vi "参数配置表.vi"() -> ()   [LabVIEW 2016, in "数据传输系统-03.lvlib"]
uses:
  <vilib>/Utility/miscctls.llb/LVPointTypeDef.ctl
  <vilib>/ptbypt/NI_PtbyPt.lvlib
panel:
  in  "参数数值":T1={"CODMn"=TRUE, "CODCr"=TRUE, "DO"=TRUE, "铜"=TRUE, "PH"=TRUE, "氨氮"=TRUE, "比电导率"=TRUE, "水温"=TRUE, "COD"=TRUE, "浊度"=TRUE, "总氮"=TRUE, "总磷"=TRUE, "叶绿素a"=TRUE, "藻密度"=TRUE, "水位"=TRUE, "流速"=TRUE, "方向"=TRUE, "瞬时流量"=TRUE, "累积流量"=TRUE, "正累积流量"=TRUE, "负累积流量"=TRUE, "亚硝氮"=TRUE, "硫化物"=TRUE, "ORP"=TRUE, "铅"=TRUE, "镉"=TRUE, "锌"=TRUE, "镍"=TRUE, "锰"=TRUE, "汞"=TRUE, "气温"=TRUE, "气压"=TRUE, "风速"=TRUE, "风向"=TRUE, "空气温度"=TRUE, "相对湿度"=TRUE, "分钟雨量"=TRUE, "小时雨量"=TRUE, "日雨量"=TRUE, "累积雨量"=TRUE, "盐度"=TRUE, "磷酸盐"=TRUE, "硝氮"=TRUE, "氟化物"=TRUE, "挥发酚"=TRUE, "氯化物"=TRUE, "蓝绿藻"=TRUE, "余氯"=TRUE, "综合生物毒性"=TRUE, "艏向"=TRUE, "横摇"=TRUE, "纵摇"=TRUE, "分层标志"=TRUE, "层状态1"=TRUE, "层状态2"=TRUE, "水平平均流速"=TRUE, "流向"=TRUE, "北向流速分量"=TRUE, "东向流速分量"=TRUE, "垂直流速分量"=TRUE, "最大波高"=TRUE, "最大波周期"=TRUE, "1/10波高"=TRUE, "1/10波周期"=TRUE, "有效波高"=TRUE, "有效波周期"=TRUE, "平均波高"=TRUE, "平均波周期"=TRUE, "波向"=TRUE, "波个数"=TRUE, "水深"=TRUE, "X轴流速"=TRUE, "Y轴流速"=TRUE, "信号强度"=TRUE, "电压"=TRUE, "悬浮物"=TRUE}
  in  "协议标准":T2(ring)
  in  "加密传输":bool
  in  "数据库类型":enum16{"Access", "SQLite"}(ring)
  in  "应用环境":T3
  in  "屏蔽维护数据":bool
  in  "数据发送延时时间/s":i32
  in  "判断数据反馈":enum16{"非严格判断", "严格判断", "不判断"}(ring)
  in  "仪器参数发送":bool
  in  "地表水/污染源":bool
  in  "间隔时间/分钟":i32
  in  "数据发送通道":enum16{"TCP", "VISA"}(ring)
  in  "数据发送协议":enum16{"2005-212协议", "2017-212协议"}(ring)=enum."2017-212协议"
  in  "数据触发上传方式":enum16{"出数即刻发送", "间隔时间发送", "整点发送"}(ring)
  in  "数据组合发送":bool
  in  "日志、参数发送":bool
  in  "2011发送":bool
  in  "返回":bool
  out "配置表格":string[][](table)
  # "因子编码，单位配置，上传功能码，小时、质控数据上传触发方式"
  # "参数配置"
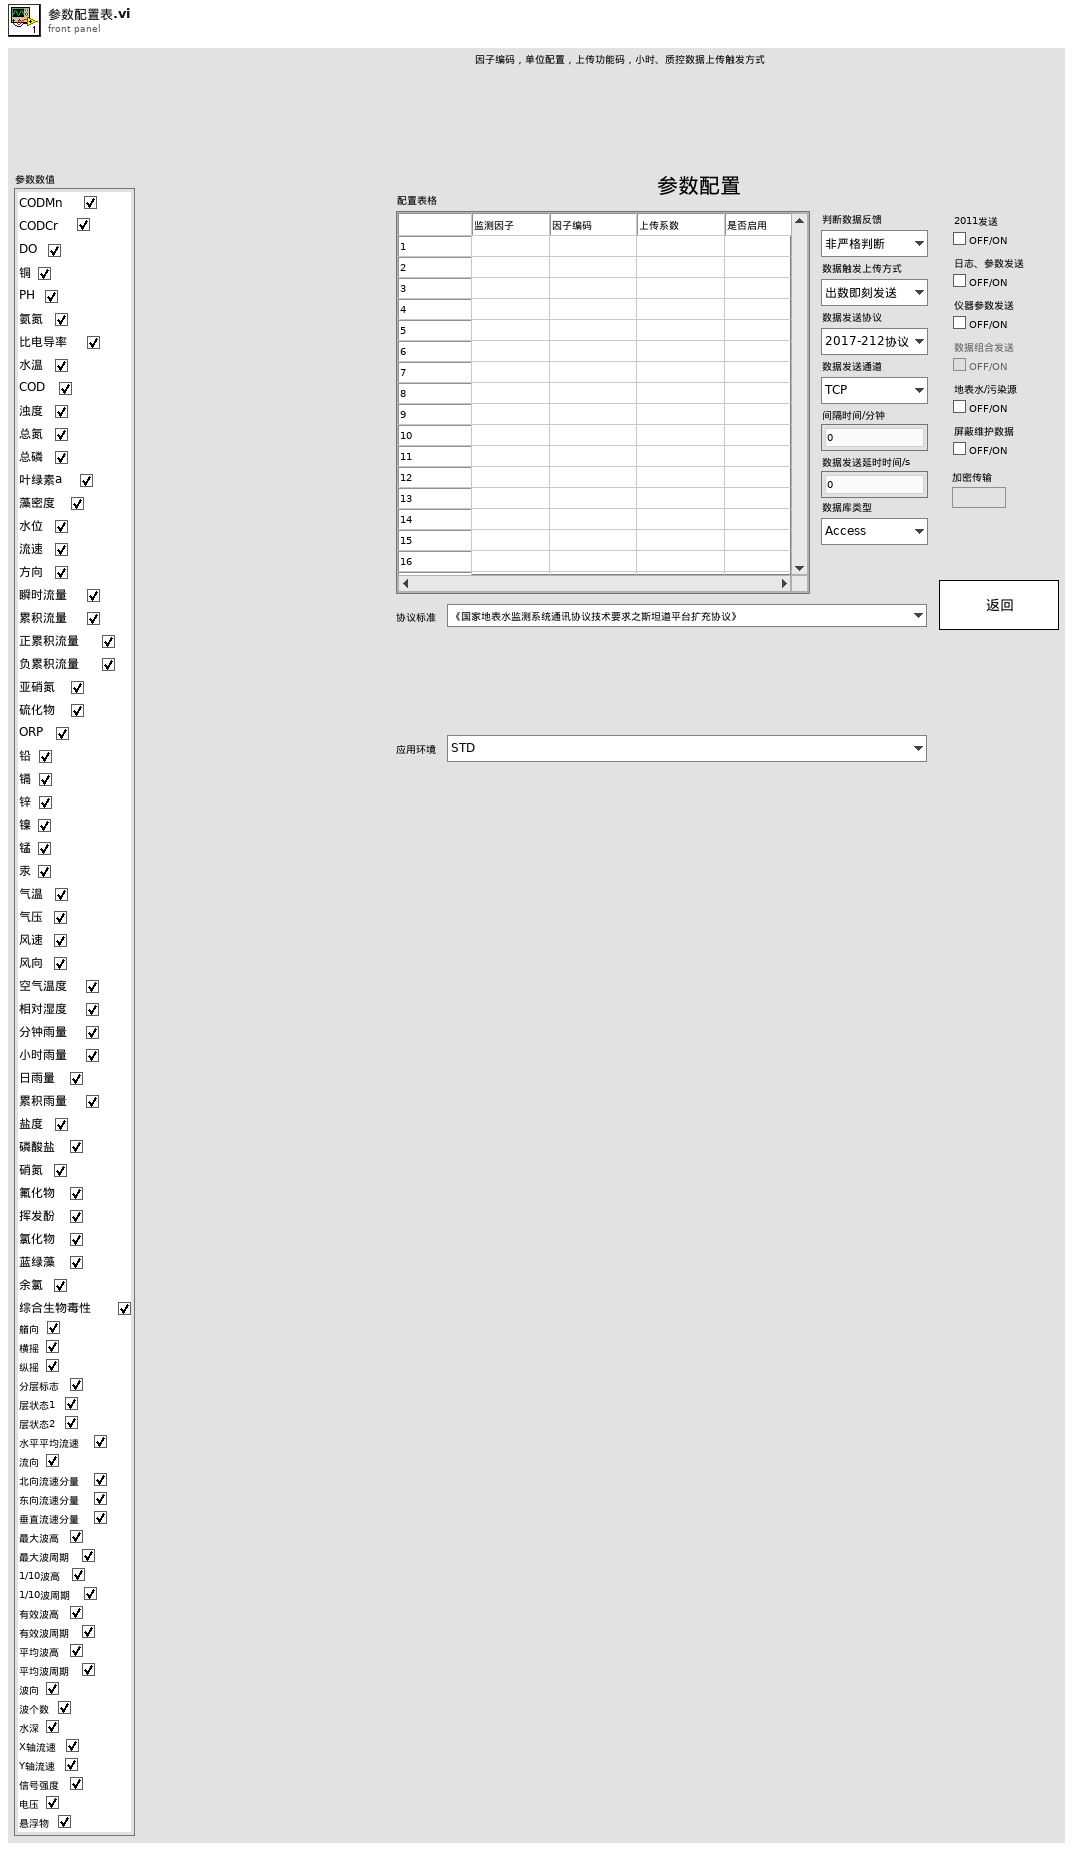
[diagram p1: front panel]
types:
  T1 = cluster{"CODMn":bool, "CODCr":bool, "DO":bool, "铜":bool, "PH":bool, "氨氮":bool, "比电导率":bool, "水温":bool, "COD":bool, "浊度":bool, "总氮":bool, "总磷":bool, "叶绿素a":bool, "藻密度":bool, "水位":bool, "流速":bool, "方向":bool, "瞬时流量":bool, "累积流量":bool, "正累积流量":bool, "负累积流量":bool, "亚硝氮":bool, "硫化物":bool, "ORP":bool, "铅":bool, "镉":bool, "锌":bool, "镍":bool, "锰":bool, "汞":bool, "气温":bool, "气压":bool, "风速":bool, "风向":bool, "空气温度":bool, "相对湿度":bool, "分钟雨量":bool, "小时雨量":bool, "日雨量":bool, "累积雨量":bool, "盐度":bool, "磷酸盐":bool, "硝氮":bool, "氟化物":bool, "挥发酚":bool, "氯化物":bool, "蓝绿藻":bool, "余氯":bool, "综合生物毒性":bool, "艏向":bool, "横摇":bool, "纵摇":bool, "分层标志":bool, "层状态1":bool, "层状态2":bool, "水平平均流速":bool, "流向":bool, "北向流速分量":bool, "东向流速分量":bool, "垂直流速分量":bool, "最大波高":bool, "最大波周期":bool, "1/10波高":bool, "1/10波周期":bool, "有效波高":bool, "有效波周期":bool, "平均波高":bool, "平均波周期":bool, "波向":bool, "波个数":bool, "水深":bool, "X轴流速":bool, "Y轴流速":bool, "信号强度":bool, "电压":bool, "悬浮物":bool}
  T2 = enum16{"《国家地表水监测系统通讯协议技术要求之斯坦道平台扩充协议》", "《国家地表水监测系统通讯协议技术要求》", "《国家地表水监测系统通讯协议技术要求之安徽皖仪省级平台扩充协议》"}
  T3 = typedef "数据传输系统-03.lvlib/应用环境.ctl" = enum16{"STD", "GB212", "婉仪平台"}
  T4 = typedef "LVPointTypeDef.ctl" = cluster{"Horizontal":i16, "Vertical":i16}
  T5 = cluster{"子数组[0]":string, "子数组[1]":string, "子数组[2]":string, "子数组[3]":string, "子数组[4]":string, "子数组[5]":string, "子数组[6]":string, "子数组[7]":string, "子数组[8]":string, "子数组[9]":string, "子数组[10]":string, "子数组[11]":string, "子数组[12]":string, "子数组[13]":string, "子数组[14]":string, "子数组[15]":string, "子数组[16]":string, "子数组[17]":string, "子数组[18]":string, "子数组[19]":string, "子数组[20]":string, "子数组[21]":string, "子数组[22]":string, "子数组[23]":string, "子数组[24]":string, "子数组[25]":string, "子数组[26]":string, "子数组[27]":string, "子数组[28]":string, "子数组[29]":string, "子数组[30]":string, "子数组[31]":string, "子数组[32]":string, "子数组[33]":string, "子数组[34]":string, "子数组[35]":string, "子数组[36]":string, "子数组[37]":string, "子数组[38]":string, "子数组[39]":string, "子数组[40]":string, "子数组[41]":string, "子数组[42]":string, "子数组[43]":string, "子数组[44]":string, "子数组[45]":string, "子数组[46]":string, "子数组[47]":string, "子数组[48]":string, "子数组[49]":string, "子数组[50]":string, "子数组[51]":string, "子数组[52]":string, "子数组[53]":string, "子数组[54]":string, "子数组[55]":string, "子数组[56]":string, "子数组[57]":string, "子数组[58]":string, "子数组[59]":string, "子数组[60]":string, "子数组[61]":string, "子数组[62]":string, "子数组[63]":string, "子数组[64]":string, "子数组[65]":string, "子数组[66]":string, "子数组[67]":string, "子数组[68]":string, "子数组[69]":string, "子数组[70]":string, "子数组[71]":string, "子数组[72]":string, "子数组[73]":string, "子数组[74]":string, "子数组[75]":string}
  T6 = enum8{"Enabled", "Disabled", "Disabled and Grayed Out"}
  T7 = typedef "LVRowAndColumnTypeDef.ctl" = cluster{"Row":i32, "Column":i32}
  T8 = cluster{"[0]":string, "[1]":string, "[2]":string, "[3]":string, "[4]":string, "[5]":string, "[6]":string, "[7]":string}
  T9 = cluster{"[0]":string, "[1]":string, "[2]":string, "[3]":string, "[4]":string, "[5]":string, "[6]":string, "[7]":string, "[8]":string, "[9]":string, "[10]":string, "[11]":string, "[12]":string, "[13]":string}
  T10 = cluster{"[0]":string, "[1]":string, "[2]":string, "[3]":string, "[4]":string, "[5]":string, "[6]":string, "[7]":string, "[8]":string, "[9]":string, "[10]":string, "[11]":string, "[12]":string, "[13]":string, "[14]":string}
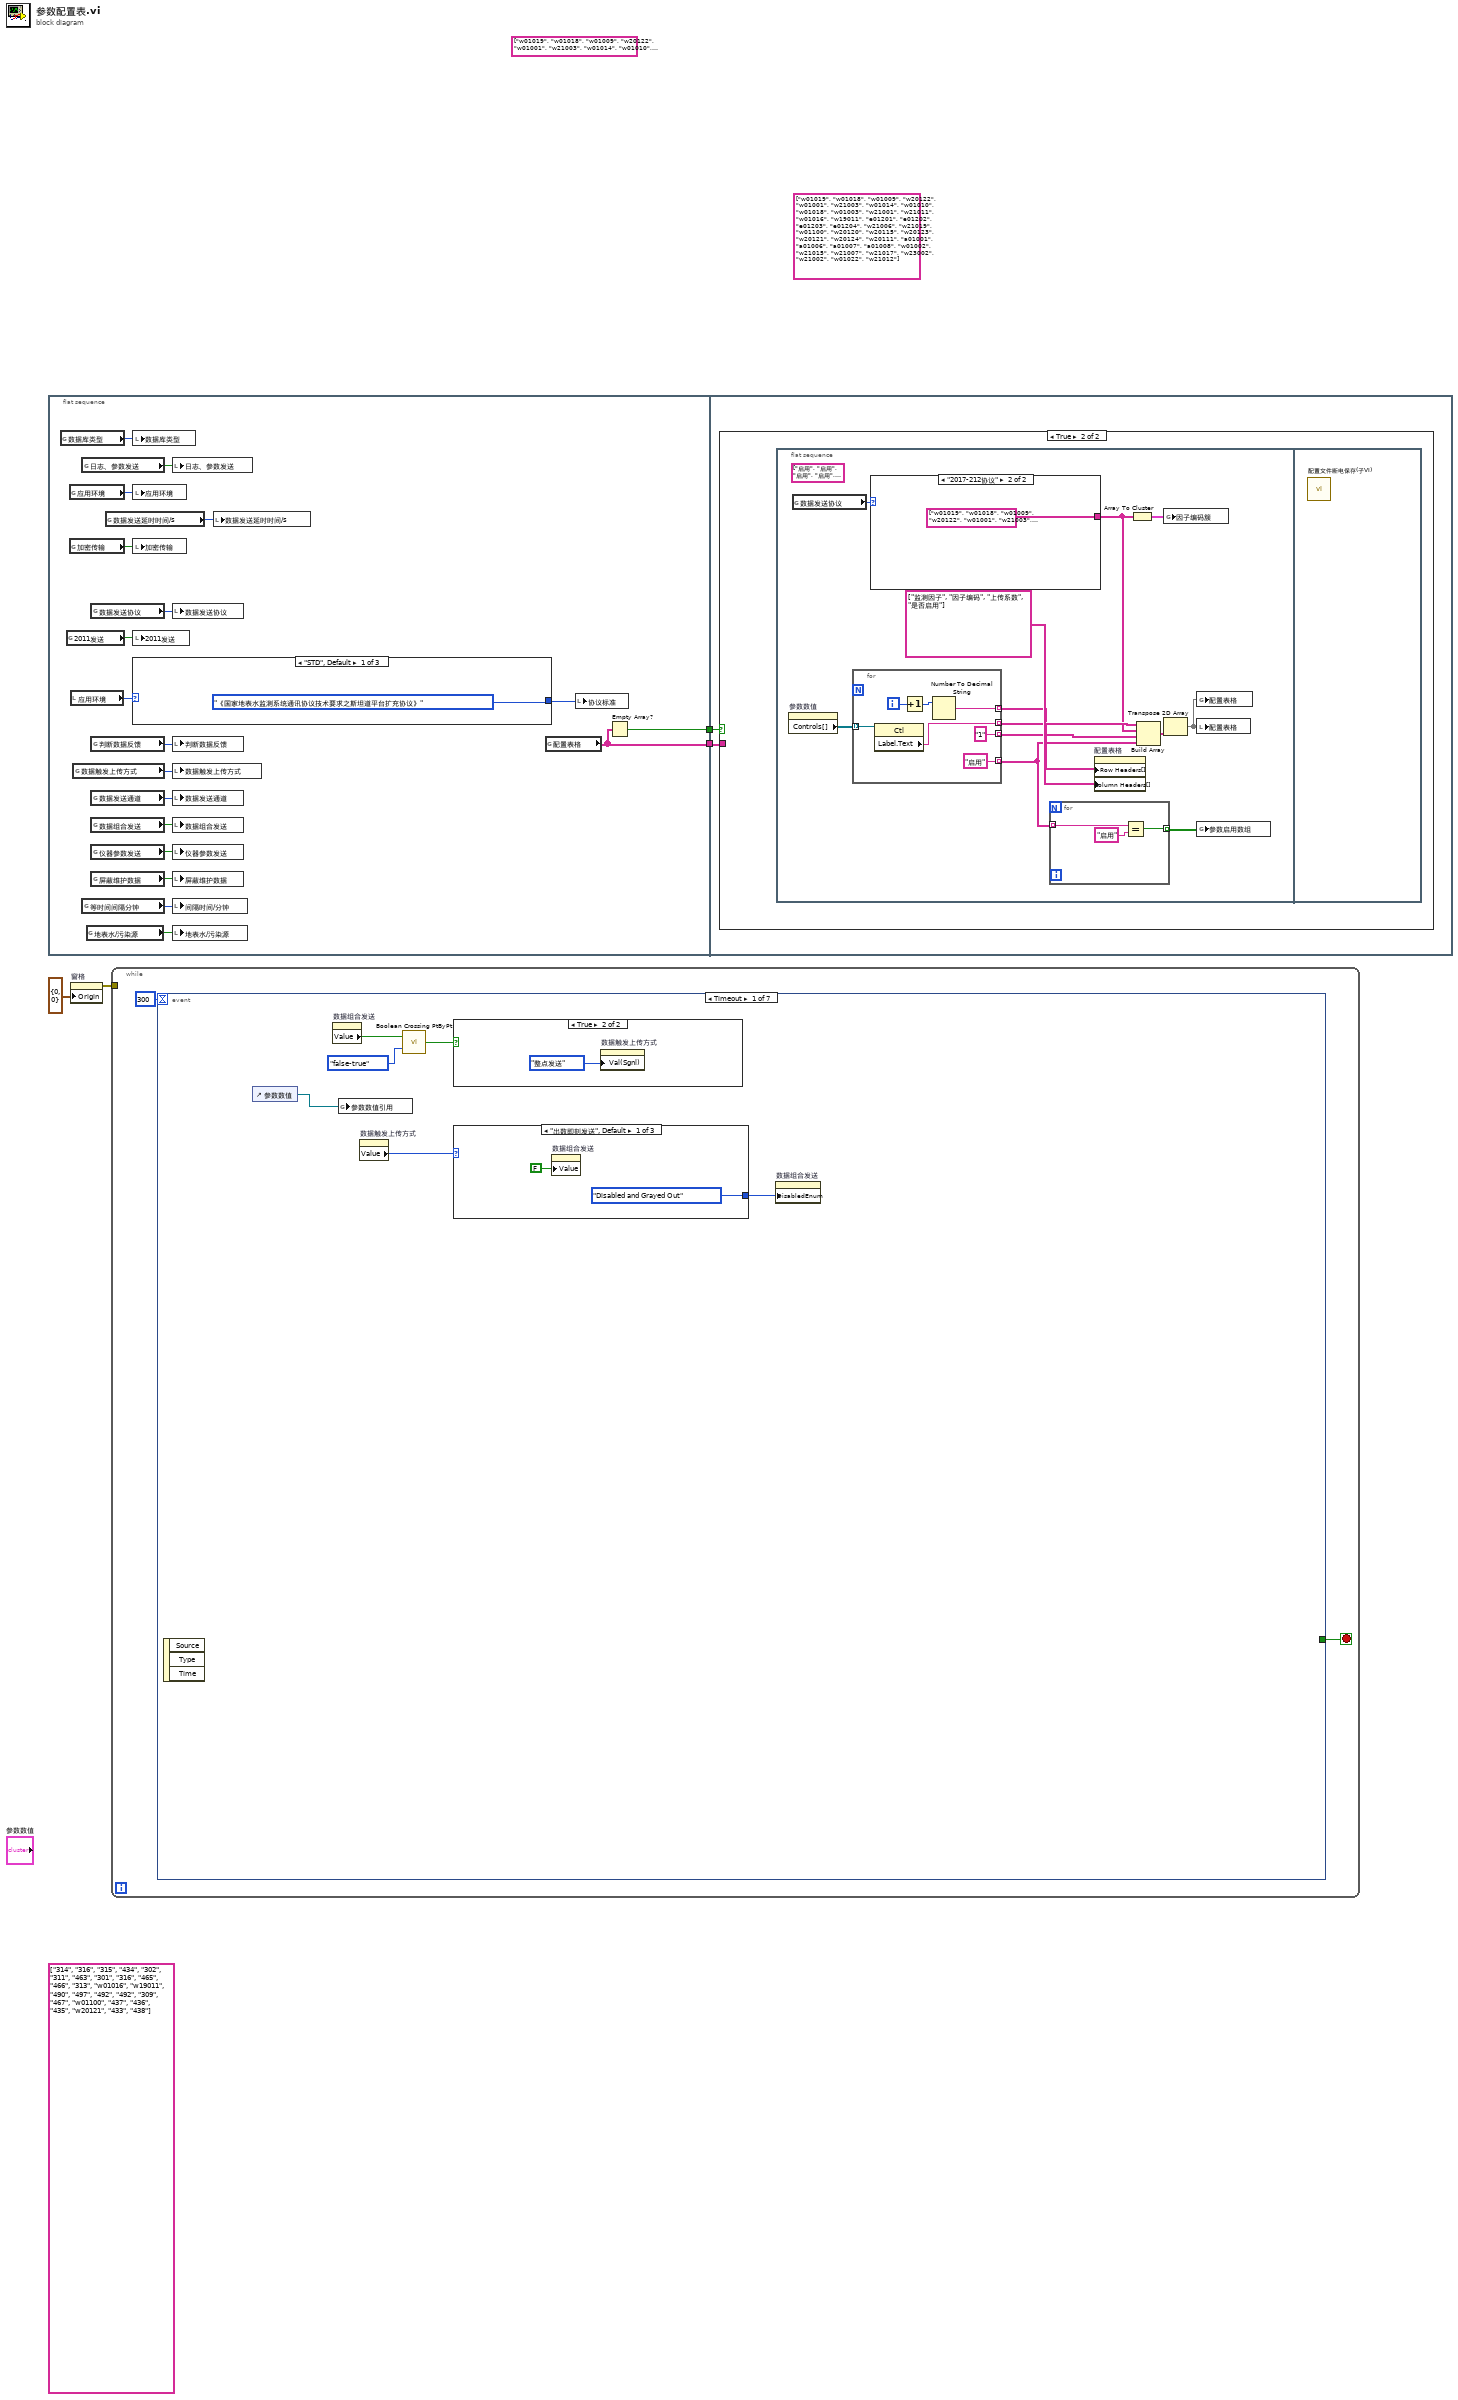
[diagram p0: block diagram]
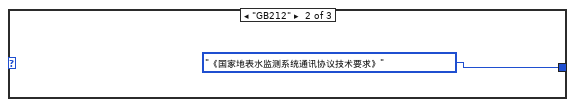
[diagram p2: hidden frame]
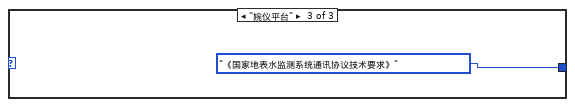
[diagram p3: hidden frame]
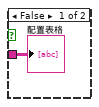
[diagram p4: hidden frame]
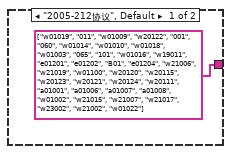
[diagram p5: hidden frame]
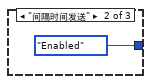
[diagram p7: hidden frame]
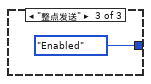
[diagram p8: hidden frame]
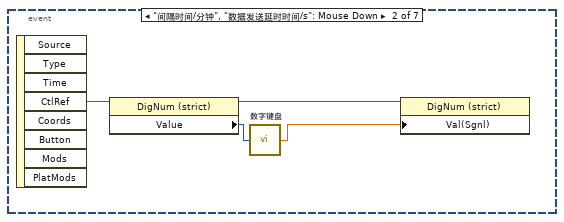
[diagram p9: hidden frame]
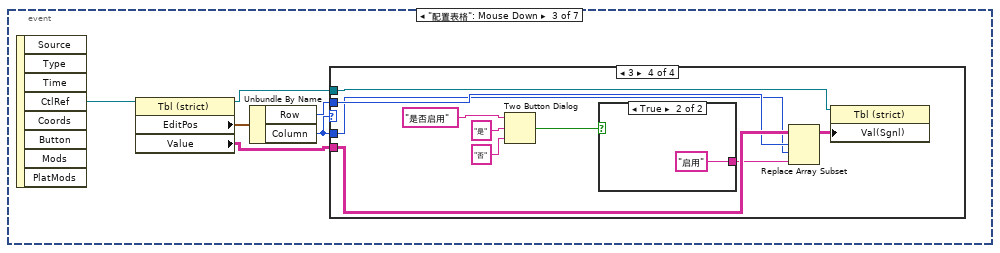
[diagram p10: hidden frame]
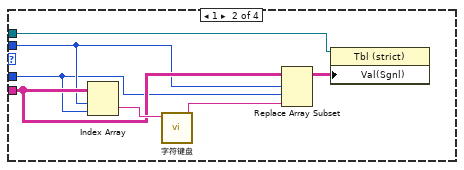
[diagram p12: hidden frame]
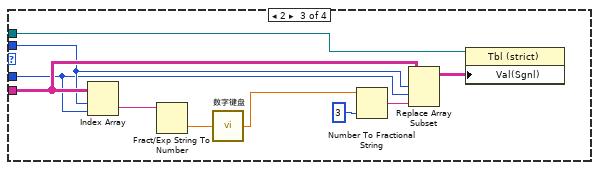
[diagram p13: hidden frame]
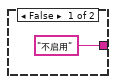
[diagram p14: hidden frame]
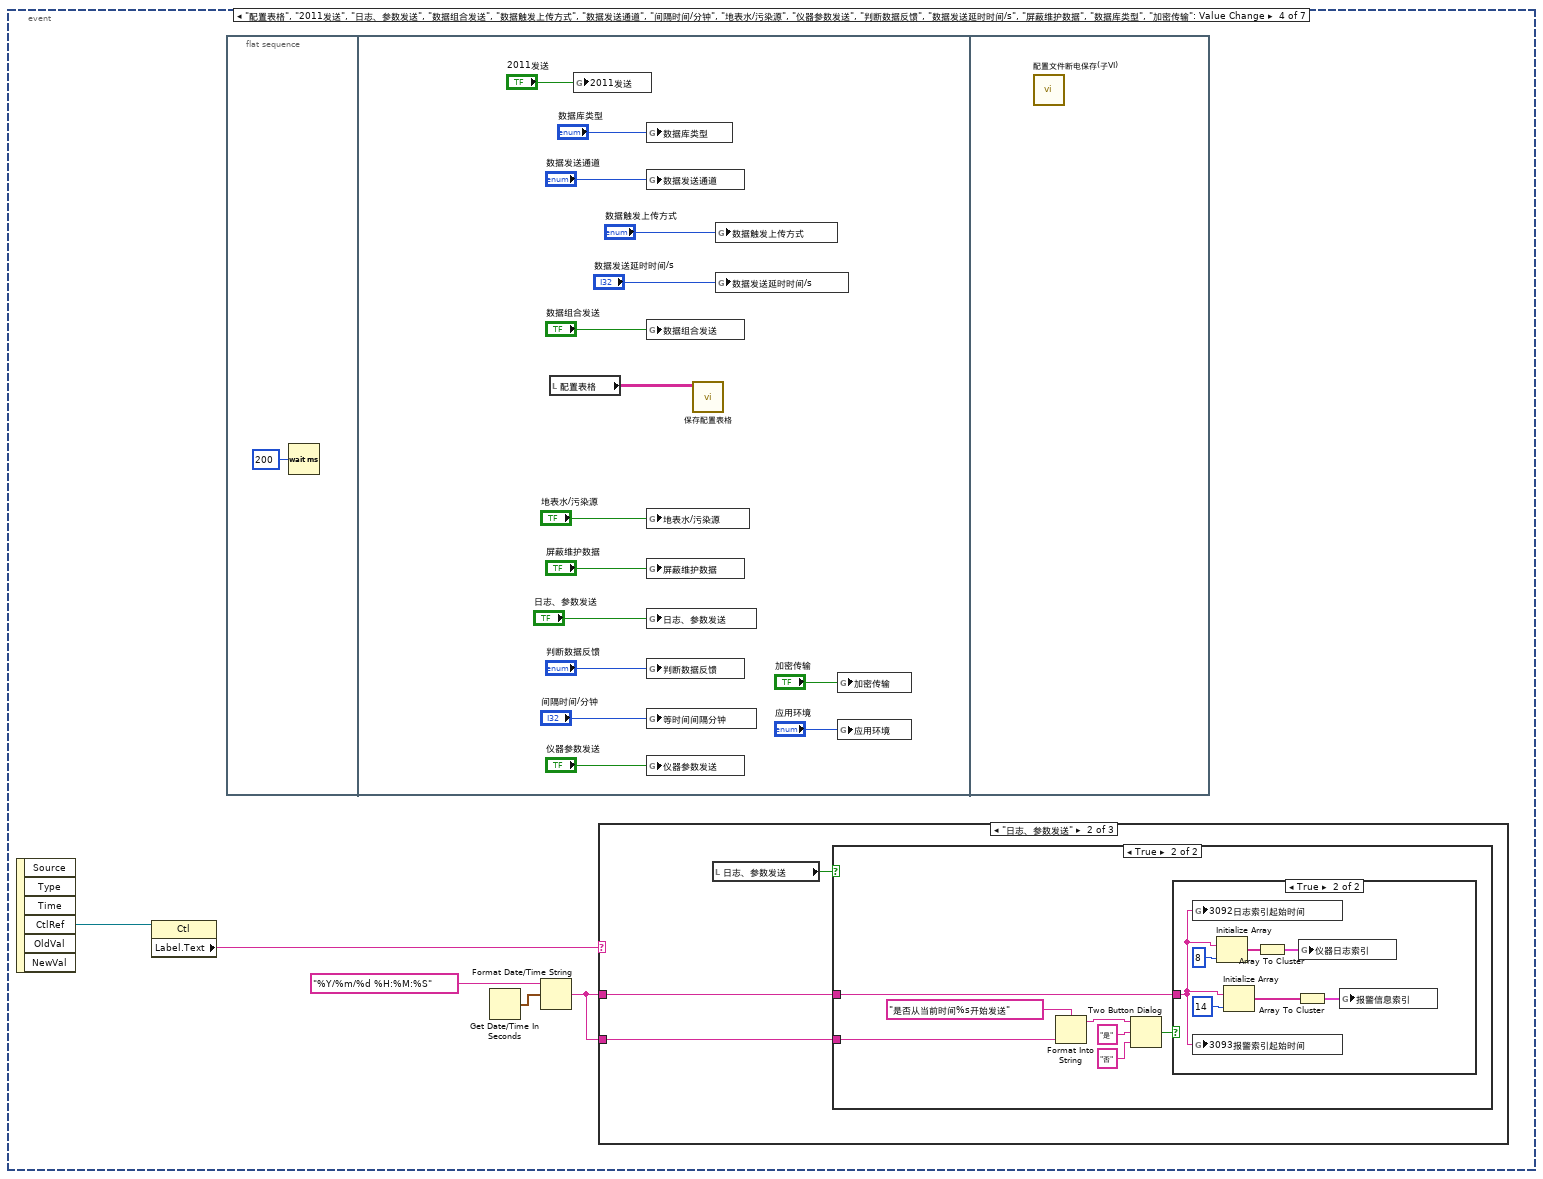
[diagram p15: hidden frame]
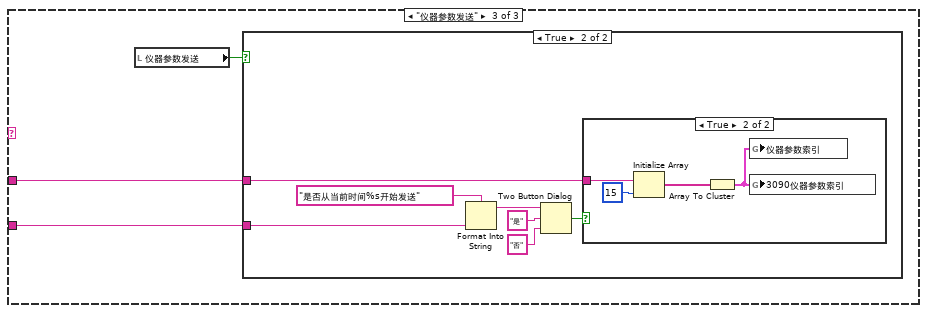
[diagram p19: hidden frame]
diagram:
  (unwired) string[] ["w01019", "w01018", "w01009", "w20122", "w01001", "w21003", "w01014", "w01010", "w01018", "w01003", "w21001", "w21011", "w01016", "w19011", "e01201", "e01202", "e01203", "e01204", "w21006", "w21019", "w01100", "w20120", "w20115", "w20123", "w20121", "w20124", "w20111", "a01001", "a01006", "a01007", "a01008", "w01002", "w21015", "w21007", "w21017", "w23002", "w21002", "w01022", "w21012"]
  (unwired) string[] ["w01019", "w01018", "w01009", "w20122", "w01001", "w21003", "w01014", "w01010", "w01018", "w01003", "w21001", "w21011", "w01016", "w19011", "e01201", "e01202", "e01203", "e01204", "w21006", "w21019", "w01100", "w20120", "w20115", "w20123", "w20121", "w20124", "w20111", "a01001", "a01006", "a01007", "a01008", "w01002", "w21015", "w21007", "w21017", "w23002", "w21002", "w01022", "w21012"]
  (unwired) string[] ["314", "316", "315", "434", "302", "311", "463", "301", "316", "465", "466", "313", "w01016", "w19011", "490", "497", "492", "492", "309", "467", "w01100", "437", "436", "435", "w20121", "433", "438"]
  n1 = flat-sequence {
    tunnel: [w5] -> w2
    tunnel: [w16] -> w1
    tunnel: w2 -> [w28]
    tunnel: w1 -> [w27]
    frame #0 {
      n2 = global read "断电保存全局.vi" "数据库类型"() -> (w9:enum16{"Access", "SQLite"})
      n3 = global read "断电保存全局.vi" "2011发送"() -> (w23:bool)
      n4 = global read "断电保存全局.vi" "应用环境"() -> (w10:T3)
      n5 = global read "断电保存全局.vi" "加密传输"() -> (w8:bool)
      n6 = local read "应用环境"() -> (w7:T3)
      n7 = global read "断电保存全局.vi" "数据触发上传方式"() -> (w19:enum16{"出数即刻发送", "间隔时间发送", "整点发送"})
      n8 = global read "断电保存全局.vi" "日志、参数发送"() -> (w21:bool)
      n9 = global read "断电保存全局.vi" "等时间间隔分钟"() -> (w15:i32)
      n10 = global read "断电保存全局.vi" "地表水/污染源"() -> (w14:bool)
      n11 = global read "断电保存全局.vi" "数据发送协议"() -> (w17:enum16{"2005-212协议", "2017-212协议"})
      n12 = global read "断电保存全局.vi" "判断数据反馈"() -> (w22:enum16{"非严格判断", "严格判断", "不判断"})
      n13 = global read "断电保存全局.vi" "数据发送通道"() -> (w18:enum16{"TCP", "VISA"})
      n14 = global read "断电保存全局.vi" "数据组合发送"() -> (w20:bool)
      n15 = global read "断电保存全局.vi" "仪器参数发送"() -> (w13:bool)
      n16 = global read "断电保存全局.vi" "屏蔽维护数据"() -> (w11:bool)
      n17 = global read "断电保存全局.vi" "数据发送延时时间/s"() -> (w12:i32)
      n18 = local write "数据库类型"(w9) -> ()
      n19 = local write "应用环境"(w10) -> ()
      n20 = local write "加密传输"(w8) -> ()
      n21 = local write "2011发送"(w23) -> ()
      n22 = case shown="\"STD\", Default" w7 {
        tunnel: [T2."《国家地表水监测系统通讯协议技术要求之斯坦道平台扩充协议》" ("协议标准") T2."《国家地表水监测系统通讯协议技术要求》" ("协议标准") T2."《国家地表水监测系统通讯协议技术要求》" ("协议标准")] -> w6
        frame "STD", Default {
        }
        frame "GB212" {
        }
        frame "婉仪平台" {
        }
      }
      n23 = local write "日志、参数发送"(w21) -> ()
      n24 = local write "数据发送协议"(w17) -> ()
      n25 = local write "判断数据反馈"(w22) -> ()
      n26 = local write "数据触发上传方式"(w19) -> ()
      n27 = local write "数据发送通道"(w18) -> ()
      n28 = local write "数据组合发送"(w20) -> ()
      n29 = local write "仪器参数发送"(w13) -> ()
      n30 = local write "屏蔽维护数据"(w11) -> ()
      n31 = local write "间隔时间/分钟"(w15) -> ()
      n32 = local write "地表水/污染源"(w14) -> ()
      n33 = local write "数据发送延时时间/s"(w12) -> ()
      n34 = global read "断电保存全局.vi" "配置表格"() -> (w16:string[][])
      n35 = local write "协议标准"(w6) -> ()
      n36 = Empty Array?(array=w16) -> (empty?=w5:bool)
    }
    frame #1 {
      n37 = case shown="True" w28 {
        tunnel: w27 -> [w29 _]
        frame False {
          "配置表格" <- w29
        }
        frame True {
          n38 = flat-sequence {
            frame #0 {
              (unwired) string[] ["启用", "启用", "启用", "启用", "启用", "启用", "启用", "启用", "启用", "启用", "启用", "启用", "启用", "启用", "启用", "启用", "启用", "启用", "启用", "启用", "启用", "启用", "启用", "启用", "启用", "启用", "启用"]
              n39 = property on="参数数值" class="Clust (strict)"() -> ("Controls[]"=w30:refnum<vi>[])  [unwired: 2 in, 2 out]
              n40 = global read "断电保存全局.vi" "数据发送协议"() -> (w32:enum16{"2005-212协议", "2017-212协议"})
              n41 = for {
                tunnel: w30 -> [w53] mode=indexing
                tunnel: [w52] -> w39 mode=indexing
                tunnel: [w50] -> w38 mode=indexing
                tunnel: ["1"] -> w35 mode=indexing
                tunnel: ["启用"] -> w33 mode=indexing
                i -> [w51]
                n42 = property class="Ctl"(reference=w53) -> ("Label.Text"=w52:string)  [unwired: 1 in, 2 out]
                n43 = Increment(x=w51) -> (x+1=w49:i32)
                n44 = Number To Decimal String(number=w49) -> (decimal integer string=w50:string)  [unwired: 1 in]
              }
              n45 = case shown="\"2017-212协议\"" w32 {
                tunnel: [string[] ["w01019", "011", "w01009", "w20122", "001", "060", "w01014", "w01010", "w01018", "w01003", "065", "101", "w01016", "w19011", "e01201", "e01202", "B01", "e01204", "w21006", "w21019", "w01100", "w20120", "w20115", "w20123", "w20121", "w20124", "w20111", "a01001", "a01006", "a01007", "a01008", "w01002", "w21015", "w21007", "w21017", "w23002", "w21002", "w01022"] string[] ["w01019", "w01018", "w01009", "w20122", "w01001", "w21003", "w01014", "w01010", "w01018", "w01003", "w21001", "w21011", "w01016", "w19011", "e01201", "e01202", "e81205", "e01203", "e01204", "e81208", "e81209", "w21006", "w21019", "w01100", "w20120", "w20115", "w20123", "w20121", "w20124", "w20111", "a01001", "e01901", "e01301", "e01302", "e01001", "e01002", "e01303", "e013031", "e013032", "e013033", "w01002", "w21015", "w21007", "w21017", "w23002", "w21002", "w01022", "w21012", "w01023", "e81216", "e81217", "e81218", "e81220", "e81221", "e81222", "e81225", "e80015", "e81223", "e81224", "e81219", "e80001", "e80002", "e80003", "e80004", "e80005", "e80006", "e80007", "e80008", "e80009", "e80016", "e81231", "e81226", "e81227", "e81228", "e81215", "w01012"] ("子数组")] -> w31
                frame "2005-212协议", Default {
                }
                frame "2017-212协议" {
                }
              }
              n46 = for {
                tunnel: w33 -> [w46] mode=indexing
                tunnel: [w44] -> w34 mode=indexing
                n47 = Equal?(x=w46, y="启用") -> (x = y?=w44:bool)
              }
              n48 = property on="配置表格" class="Tbl (strict)"("Row Headers[]"=w38, "Column Headers[]"=string[] ["监测因子", "因子编码", "上传系数", "是否启用"]) -> ()  [unwired: 2 in, 2 out]
              n49 = Array To Cluster(array=w31) -> (cluster=w36:T5)
              n50 = Build Array(w39, w31, w35, w33) -> (w41:string[][])
              n51 = global write "断电保存全局.vi" "因子编码簇"(w36) -> ()
              n52 = Transpose 2D Array(2D array=w41) -> (transposed array=w37:string[][])
              n53 = global write "断电保存全局.vi" "配置表格"(w37) -> ()
              n54 = local write "配置表格"(w37) -> ()
              n55 = global write "断电保存全局.vi" "参数启用数组"(w34) -> ()
            }
            frame #1 {
              n56 = call "配置文件断电保存(子VI).vi"() -> ()  [unwired: 12 in]
            }
          }
        }
      }
    }
  }
  n57 = property on="窗格" class="Pane"("Origin"=T4 {"Horizontal"=0, "Vertical"=0} ("原点")) -> (error out=w4:errorcluster)  [unwired: 2 in, 1 out]
  n58 = while {
    tunnel: w4 -> [_]
    stop <- w54 stop-if-true
    n59 = event shown="[0] Timeout" {
      selector: _ -> [_ _ _ _ _ _ _]
      dyn-events: _ -> [_ _ _ _ _ _ _]
      timeout: 300 -> [_ _ _ _ _ _ _]
      tunnel: [_ _ _ _ _ _ TRUE] -> w54
      event Timeout {
        n60 = event-data() -> ()  [unwired: 1 in, 3 out]
        n61 = control-ref of="参数数值"() -> (w56:refnum<vi>)
        n62 = property on="数据组合发送" class="Bool (strict)"() -> ("Value"=w59:bool)  [unwired: 2 in, 2 out]
        n63 = global write "断电保存全局.vi" "参数数值引用"(w56) -> ()
        n64 = property on="数据触发上传方式" class="Enum (strict)"() -> ("Value"=w61:enum16{"出数即刻发送", "间隔时间发送", "整点发送"})  [unwired: 2 in, 2 out]
        n65 = call <vilib>:"Boolean Crossing PtByPt.vi"("direction"=enum16{"either", "false-true", "true-false"}."false-true", "input"=w59) -> ("crossing"=w57:bool)  [unwired: 1 in]
        n66 = case shown="True" w57 {
          frame False {
          }
          frame True {
            n67 = property on="数据触发上传方式" class="Enum (strict)"("Val(Sgnl)"=enum16{"出数即刻发送", "间隔时间发送", "整点发送"}."整点发送" ("值(信号)")) -> ()  [unwired: 2 in, 2 out]
          }
        }
        n68 = case shown="\"出数即刻发送\", Default" w61 {
          tunnel: [T6."Disabled and Grayed Out" ("禁用") T6."Enabled" ("禁用") T6."Enabled" ("禁用")] -> w60
          frame "出数即刻发送", Default {
            n69 = property on="数据组合发送" class="Bool (strict)"("Value"=FALSE ("值(信号)")) -> ()  [unwired: 2 in, 2 out]
          }
          frame "间隔时间发送" {
          }
          frame "整点发送" {
          }
        }
        n70 = property on="数据组合发送" class="Bool (strict)"("DisabledEnum"=w60) -> ()  [unwired: 2 in, 2 out]
      }
      event "间隔时间/分钟", "数据发送延时时间/s": Mouse Down {
        n71 = event-data() -> ("CtlRef"=w70:refnum<vi>)  [unwired: 1 in, 7 out]
        n72 = property class="DigNum (strict)"(reference=w70) -> (reference out=w68:refnum<vi>, "Value"=w69:i32)  [unwired: 1 in, 1 out]
        n73 = call "数字键盘.vi"("OldNumber"=w69) -> ("NewNumber"=w67:sgl)
        n74 = property class="DigNum (strict)"(reference=w68, "Val(Sgnl)"=w67) -> ()  [unwired: 1 in, 2 out]
      }
      event "配置表格": Mouse Down {
        n75 = event-data() -> ("CtlRef"=w76:refnum<vi>)  [unwired: 1 in, 7 out]
        n76 = property class="Tbl (strict)"(reference=w76) -> (reference out=w72:refnum<vi>, "EditPos"=w75:T7, "Value"=w74:string[][])  [unwired: 1 in, 1 out]
        n77 = Unbundle By Name(w75) -> ("Row"=w73:i32, "Column"=w71:i32)
        n78 = case shown="3" w71 {
          tunnel: w74 -> [_ w82 w93 w97]
          tunnel: w73 -> [_ w81 w92 w96]
          tunnel: w71 -> [_ w80 w91 w95]
          tunnel: w72 -> [_ w78 w90 w98]
          frame 0, Default {
          }
          frame 1 {
            n79 = Index Array(array=w82, index (row)=w81, index (col)=w80) -> (element=w83:string)
            n80 = call "字符键盘.vi"("原值"=w83) -> ("x+y"=w79:string)  [unwired: 10 in]
            n81 = Replace Array Subset(array=w82, new element=w79, index (row)=w81, index (col)=w80) -> (w77:string[][])
            n82 = property class="Tbl (strict)"(reference=w78, "Val(Sgnl)"=w77) -> ()  [unwired: 1 in, 2 out]
          }
          frame 2 {
            n83 = Index Array(array=w93, index (row)=w92, index (col)=w91) -> (element=w88:string)
            n84 = Fract/Exp String To Number(string=w88) -> (number=w87:dbl)  [unwired: 3 in, 1 out]
            n85 = call "数字键盘.vi"("OldNumber"=w87) -> ("NewNumber"=w86:sgl)
            n86 = Number To Fractional String(number=w86, precision (6)=i16 3 ("精度(6)")) -> (F-format string=w85:string)  [unwired: 2 in]
            n87 = Replace Array Subset(array=w93, new element=w85, index (row)=w92, index (col)=w91) -> (w89:string[][])
            n88 = property class="Tbl (strict)"(reference=w90, "Val(Sgnl)"=w89) -> ()  [unwired: 1 in, 2 out]
          }
          frame 3 {
            n89 = Two Button Dialog(message="是否启用" ("消息"), 1:"否" ("F按钮名称（“取消”）"), 2:"是" ("T按钮名称（“确定”）")) -> (T button?=w100:bool)
            n90 = case shown="True" w100 {
              tunnel: ["不启用" "启用"] -> w94
              frame False {
              }
              frame True {
              }
            }
            n91 = Replace Array Subset(array=w97, new element=w94, index (row)=w96, index (col)=w95) -> (w99:string[][])
            n92 = property class="Tbl (strict)"(reference=w98, "Val(Sgnl)"=w99) -> ()  [unwired: 1 in, 2 out]
          }
        }
      }
      event "配置表格", "2011发送", "日志、参数发送", "数据组合发送", "数据触发上传方式", "数据发送通道", "间隔时间/分钟", "地表水/污染源", "仪器参数发送", "判断数据反馈", "数据发送延时时间/s", "屏蔽维护数据", "数据库类型", "加密传输": Value Change {
        n93 = event-data() -> ("CtlRef"=w110:refnum<vi>)  [unwired: 1 in, 5 out]
        n94 = property class="Ctl"(reference=w110) -> ("Label.Text"=w109:string)  [unwired: 1 in, 2 out]
        n95 = flat-sequence {
          frame #0 {
            n96 = Wait (ms)(milliseconds to wait=u32 200 ("等待时间（毫秒）")) -> ()  [unwired: 1 out]
          }
          frame #1 {
            n97 = local read "配置表格"() -> (w143:string[][])
            n98 = global write "断电保存全局.vi" "2011发送"("2011发送") -> ()
            n99 = global write "断电保存全局.vi" "数据库类型"("数据库类型") -> ()
            n100 = global write "断电保存全局.vi" "数据发送通道"("数据发送通道") -> ()
            n101 = global write "断电保存全局.vi" "数据组合发送"("数据组合发送") -> ()
            n102 = global write "断电保存全局.vi" "地表水/污染源"("地表水/污染源") -> ()
            n103 = global write "断电保存全局.vi" "屏蔽维护数据"("屏蔽维护数据") -> ()
            n104 = global write "断电保存全局.vi" "日志、参数发送"("日志、参数发送") -> ()
            n105 = global write "断电保存全局.vi" "判断数据反馈"("判断数据反馈") -> ()
            n106 = global write "断电保存全局.vi" "等时间间隔分钟"("间隔时间/分钟") -> ()
            n107 = global write "断电保存全局.vi" "仪器参数发送"("仪器参数发送") -> ()
            n108 = call "保存配置表格.vi"("配置表格"=w143) -> ()  [unwired: 11 in]
            n109 = global write "断电保存全局.vi" "数据触发上传方式"("数据触发上传方式") -> ()
            n110 = global write "断电保存全局.vi" "数据发送延时时间/s"("数据发送延时时间/s") -> ()
            n111 = global write "断电保存全局.vi" "加密传输"("加密传输") -> ()
            n112 = global write "断电保存全局.vi" "应用环境"("应用环境") -> ()
          }
          frame #2 {
            n113 = call "配置文件断电保存(子VI).vi"() -> ()  [unwired: 12 in]
          }
        }
        n114 = Get Date/Time In Seconds() -> (seconds since 1Jan1904=w108:timestamp)
        n115 = Format Date/Time String(time format string (%c)="%Y/%m/%d %H:%M:%S" ("时间格式字符串(%c)"), seconds (now)=w108) -> (date/time string=w106:string)  [unwired: 1 in]
        n116 = case shown="\"日志、参数发送\"" w109 {
          tunnel: w106 -> [_ w112 w129]
          tunnel: w106 -> [_ w111 w128]
          frame "假", Default {
          }
          frame "日志、参数发送" {
            n117 = local read "日志、参数发送"() -> (w113:bool)
            n118 = case shown="True" w113 {
              tunnel: w112 -> [_ w117]
              tunnel: w111 -> [_ w115]
              frame False {
              }
              frame True {
                n119 = Format Into String(format string="是否从当前时间%s开始发送" ("消息"), w115) -> (resulting string=w114:string)  [unwired: 2 in, 1 out]
                n120 = Two Button Dialog(message=w114, 1:"否" ("F按钮名称（“取消”）"), 2:"是" ("T按钮名称（“确定”）")) -> (T button?=w118:bool)
                n121 = case shown="True" w118 {
                  tunnel: w117 -> [_ w121]
                  frame False {
                  }
                  frame True {
                    n122 = global write "全局 时间2.vi" "3092日志索引起始时间"(w121) -> ()
                    n123 = global write "全局 时间2.vi" "3093报警索引起始时间"(w121) -> ()
                    n124 = Initialize Array(w121, 8 ("维数大小")) -> (w122:string[])
                    n125 = Initialize Array(w121, 14 ("维数大小")) -> (w125:string[])
                    n126 = Array To Cluster(array=w122) -> (cluster=w123:T8)
                    n127 = Array To Cluster(array=w125) -> (cluster=w124:T9)
                    n128 = global write "全局 时间2.vi" "仪器日志索引"(w123) -> ()
                    n129 = global write "全局 时间2.vi" "报警信息索引"(w124) -> ()
                  }
                }
              }
            }
          }
          frame "仪器参数发送" {
            n130 = local read "仪器参数发送"() -> (w130:bool)
            n131 = case shown="True" w130 {
              tunnel: w129 -> [_ w134]
              tunnel: w128 -> [_ w132]
              frame False {
              }
              frame True {
                n132 = Format Into String(format string="是否从当前时间%s开始发送" ("消息"), w132) -> (resulting string=w131:string)  [unwired: 2 in, 1 out]
                n133 = Two Button Dialog(message=w131, 1:"否" ("F按钮名称（“取消”）"), 2:"是" ("T按钮名称（“确定”）")) -> (T button?=w135:bool)
                n134 = case shown="True" w135 {
                  tunnel: w134 -> [_ w139]
                  frame False {
                  }
                  frame True {
                    n135 = Initialize Array(w139, 15 ("维数大小")) -> (w141:string[])
                    n136 = Array To Cluster(array=w141) -> (cluster=w138:T10)
                    n137 = global write "全局 时间2.vi" "仪器参数索引"(w138) -> ()
                    n138 = global write "全局 时间2.vi" "3090仪器参数索引"(w138) -> ()
                  }
                }
              }
            }
          }
        }
      }
      event "数据发送协议": Value Change {
        (unwired) string[] ["w01019", "w01018", "w01009", "w20122", "w01001", "w21003", "w01014", "w01010", "w01018", "w01003", "w21001", "w21011", "w01016", "w19011", "e01201", "e01202", "e01203", "e01204", "w21006", "w21019", "w01100", "w20120", "w20115", "w20123", "w20121", "w20124", "w20111", "a01001", "a01006", "a01007", "a01008", "w01002", "w21015", "w21007", "w21017", "w23002", "w21002", "w01022", "w21024"]
        n139 = event-data() -> ()  [unwired: 1 in, 6 out]
        n140 = flat-sequence {
          frame #0 {
            n141 = global write "断电保存全局.vi" "数据发送协议"("数据发送协议") -> ()
            n142 = case shown="\"2017-212协议\"" "数据发送协议" {
              tunnel: [string[] ["w01019", "011", "w01009", "w20122", "001", "060", "w01014", "w01010", "w01018", "w01003", "065", "101", "w01016", "w19011", "e01201", "e01202", "B01", "e01204", "w21006", "w21019", "w01100", "w20120", "w20115", "w20123", "w20121", "w20124", "w20111", "a01001", "a01006", "a01007", "a01008", "w01002", "w21015", "w21007", "w21017", "w23002", "w21002", "w01022"] string[] ["w01019", "w01018", "w01009", "w20122", "w01001", "w21003", "w01014", "w01010", "w01018", "w01003", "w21001", "w21011", "w01016", "w19011", "e01201", "e01202", "e01203", "e01204", "w21006", "w21019", "w01100", "w20120", "w20115", "w20123", "w20121", "w20124", "w20111", "a01001", "e01901", "e01301", "e01302", "e01001", "e01002", "e01303", "e013031", "e013032", "e013033", "w01002", "w21015", "w21007", "w21017", "w23002", "w21002", "w01022", "w21012"] ("添加的数组")] -> w158
              frame "2005-212协议", Default {
              }
              frame "2017-212协议" {
              }
            }
            n143 = local read "配置表格"() -> (w162:string[][])
            n144 = Replace Array Subset(array=w162, new element=w158, index (col)=1 ("禁用的索引 (列)")) -> (w160:string[][])  [unwired: 1 in]
            n145 = property on="配置表格" class="Tbl (strict)"("Val(Sgnl)"=w160) -> ()  [unwired: 2 in, 2 out]
            n146 = global write "断电保存全局.vi" "配置表格"(w160) -> ()
          }
          frame #1 {
            n147 = call "配置文件断电保存(子VI).vi"() -> ()  [unwired: 12 in]
          }
        }
      }
      event "协议标准": Value Change {
        n148 = event-data() -> ()  [unwired: 1 in, 6 out]
        n149 = case shown="\"《国家地表水监测系统通讯协议技术要求之斯坦道平台扩充协议》\", Default" "协议标准" {
          tunnel: [应用环境."STD" ("值(信号)") 应用环境."GB212" ("值(信号)") 应用环境."婉仪平台" ("值(信号)")] -> w165
          frame "《国家地表水监测系统通讯协议技术要求之斯坦道平台扩充协议》", Default {
          }
          frame "《国家地表水监测系统通讯协议技术要求》" {
          }
          frame "《国家地表水监测系统通讯协议技术要求之安徽皖仪省级平台扩充协议》" {
          }
        }
        n150 = property on="应用环境" class="Enum (strict)"("Val(Sgnl)"=w165) -> ()  [unwired: 2 in, 2 out]
      }
      event "返回": Value Change; Panel Close {
        n151 = event-data() -> ()  [unwired: 1 in, 3 out]
      }
    }
  }
